vi "Read Depthed_.vi"(8 "error in (no error)":errorcluster, 11 "Video Frame in":refnum<class "Video Frame.lvclass">) -> (0 "error out":errorcluster, 2 "Depthed?":bool, 3 "Video Frame out":refnum<class "Video Frame.lvclass">)   [LabVIEW 2018, in "Video Frame.lvclass"]
uses:
  Video Frame.lvclass
  Video Frame.lvclass/Video Frame.ctl
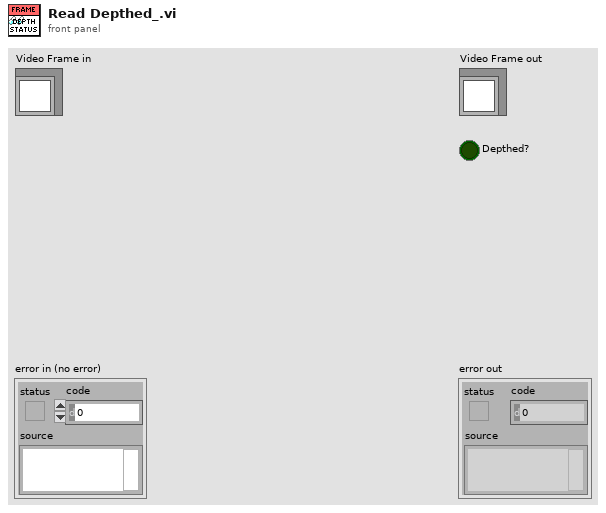
[diagram p1: front panel]
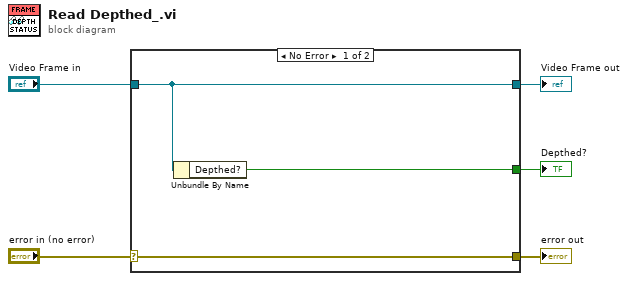
[diagram p0: block diagram]
diagram:
  n1 = case shown="No Error" "error in (no error)" {
    selector: "error in (no error)" -> [w8 w9]
    tunnel: [w8 w9] -> w4
    tunnel: [w7 w10] -> w2
    tunnel: "Video Frame in" -> [w7 w10]
    tunnel: [w6 _] -> w1
    frame No Error {
      n2 = Unbundle By Name(w7) -> ("Depthed?"=w6:bool)
    }
    frame Error {
    }
  }
  "error out" <- w4
  "Video Frame out" <- w2
  "Depthed?" <- w1
